vi "Mode 1 - GUI.vi"() -> ()   [LabVIEW 2020]
uses:
  <vilib>/Platform/TimedLoop/XDataNode/timing_clust.ctl
  <vilib>/Platform/TimedLoop/XDataNode/nitl_modes.ctl
  <vilib>/Platform/TimedLoop/XDataNode/wakeup.ctl
  <vilib>/Instr/_visa.llb/VISA Configure Serial Port (Instr).vi
  <vilib>/platform/TimedLoop/XDataNode/XDataNode.xnode
  <vilib>/Platform/TimedLoop/XDataNode/XDNodeRunTimeDep.lvlib
panel:
  in  "byte count":u32=31
  out "Counter Up ?":bool
  in  "Slider 2 Counter":i32
  in  "Slider 1 Counter":i32
  out "Black Workpiece":bool
  out "White Workpiece":bool
  in  "STOP":bool
  in  "VISA resource name":refnum<visa-resource-name>
  out "Report Data":string
  # "TRAINER ARDUINO\nMPS SORTING STATION"
  # "Mechatronics Engineering 2nd Generation\n  Vocational High School 2 Bojonegoro\n2021"
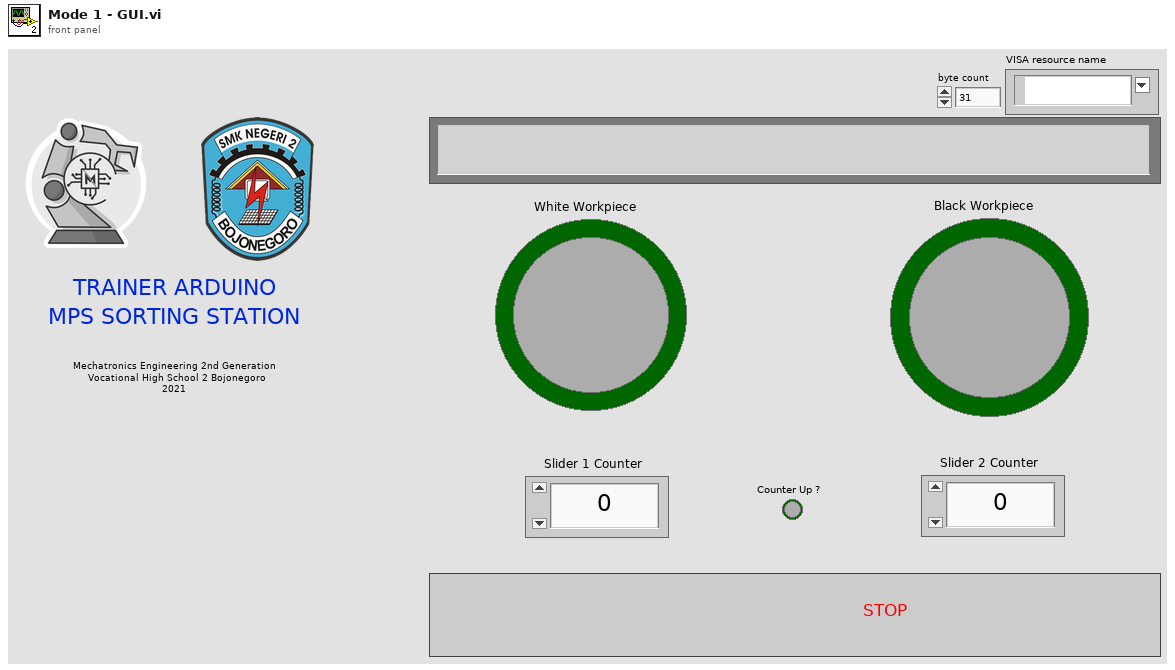
[diagram p1: front panel]
types:
  T1 = typedef "XDNodeRunTimeDep.lvlib/timing_clust.ctl" = cluster{"Expected End [f-1]":u64, "Actual End [f-1]":u64, "Finished Late? [f-1]":bool, "Expected End [i-1]":u64, "Actual End [i-1]":u64, "Finished Late? [i-1]":bool, "Expected Start [i]":u64, "Actual Start [i]":u64, "Expected Start [f]":u64, "Actual Start [f]":u64, "Source Name":string, "Structure Name":string, "Period":i64, "Deadline":i64, "Offset":i64, "Start":i64, "Priority":i32, "Timeout":i32, "Mode":T2, "Wakeup Reason":T3, "Error":errorcluster, "Source Type":string, "Secondary Source Type":string, "Global End Time":u64, "Global Start Time":u64, "Frame Duration":u64, "Iteration Duration":u64, "Assigned CPU":i32, "I/O Scan Engine Mode":u32}
  T2 = typedef "XDNodeRunTimeDep.lvlib/nitl_modes.ctl" = enum32{"No Change", "Process missed periods, maintain original phase", "Discard missed periods, maintain original phase", "Process missed periods, ignore original phase", "Discard missed periods, ignore original phase"}
  T3 = typedef "XDNodeRunTimeDep.lvlib/wakeup.ctl" = enum32{"Normal", "Aborted", "Asynchronous wakeup", "Timing source error", "Timed loop error", "Timeout"}
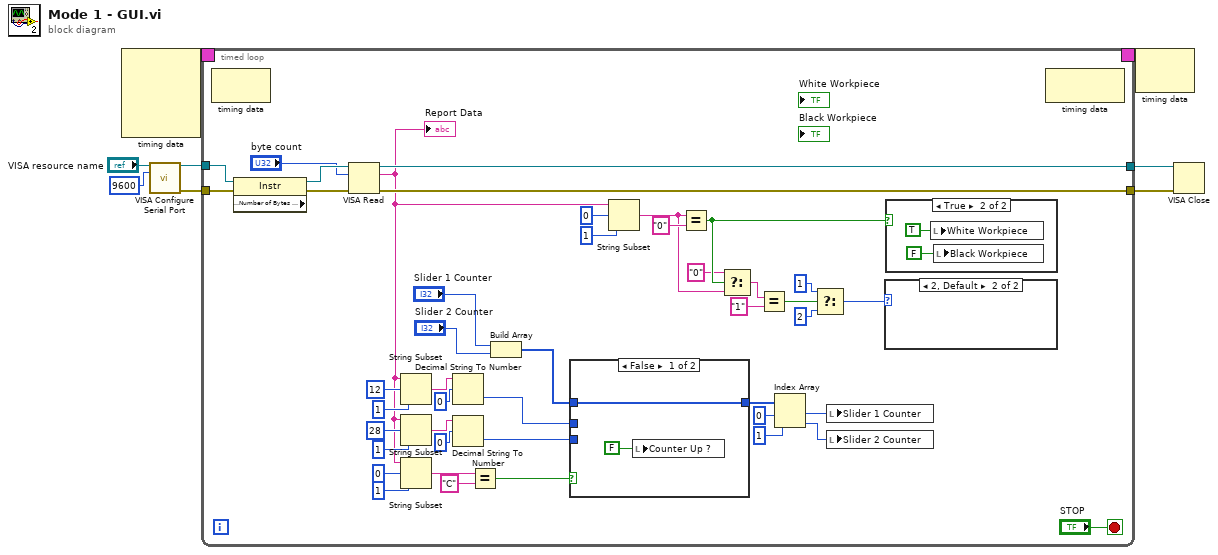
[diagram p0: block diagram]
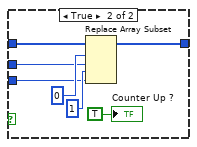
[diagram p2: hidden frame]
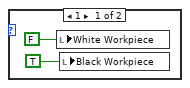
[diagram p3: hidden frame]
diagram:
  n1 = node-c288() -> (w8:T1)  [unwired: 4 in]
  n2 = call-poly "VISA Configure Serial Port"("VISA resource name"="VISA resource name", "baud rate (9600)"=u32 9600) -> ("VISA resource name out"=w6:refnum<visa-resource-name>, "error out"=w5:errorcluster)  [unwired: 12 in]
  n3 = timed-loop {
    timing: w8 -> [_]
    timing-out: [_] -> w7
    tunnel: w6 -> [w52]
    tunnel: w5 -> [w51]
    tunnel: [w48] -> w4
    tunnel: [w47] -> w3
    stop <- "STOP" stop-if-true
    n4 = node-c288() -> ()  [unwired: 1 in, 1 out]
    n5 = property class="Instr" props=["Serial Settings:Number of Bytes at Serial Port"](reference=w52, error in=w51) -> (reference out=w50:refnum<visa-resource-name>, error out=w49:errorcluster)  [unwired: 1 out]
    n6 = VISA Read(VISA resource name=w50, byte count="byte count", error in (no error)=w49) -> (VISA resource name out=w48:refnum<visa-resource-name>, read buffer=w9:string, error out=w47:errorcluster)  [unwired: 1 out]
    "Report Data" <- w9
    n7 = String Subset(string=w9, offset (0)=12, length (rest)=1 ("length (rest)")) -> (substring=w25:string)
    n8 = String Subset(string=w9, offset (0)=28, length (rest)=1 ("length (rest)")) -> (substring=w26:string)
    n9 = String Subset(string=w9, offset (0)=0, length (rest)=1 ("length (rest)")) -> (substring=w29:string)
    n10 = Decimal String To Number(string=w25, offset=0) -> (number=w22:i32)  [unwired: 1 in, 1 out]
    n11 = Decimal String To Number(string=w26, offset=0) -> (number=w21:i32)  [unwired: 1 in, 1 out]
    n12 = Equal?(x=w29, y="C") -> (x = y?=w27:bool)
    n13 = Build Array("Slider 1 Counter", "Slider 2 Counter") -> (w20:i32[])
    n14 = case shown="False" w27 {
      tunnel: w22 -> [_ w59]
      tunnel: w21 -> [_ w58]
      tunnel: w20 -> [w54 w57]
      tunnel: [w54 w56] -> w19
      frame False {
        n15 = local write "Counter Up ?"(FALSE ("Boolean")) -> ()
      }
      frame True {
        n16 = Replace Array Subset(array=w57, new element #1=w59, index #1=0 ("index"), new element #2=w58, index #2=1 ("index")) -> (w56:i32[])
        "Counter Up ?" <- TRUE ("Boolean")
      }
    }
    n17 = String Subset(string=w9, offset (0)=0, length (rest)=1 ("length (rest)")) -> (substring=w10:string)
    n18 = Equal?(x=w10, y="0") -> (x = y?=w43:bool)
    n19 = Select(t="0" ("y"), s=w43, f=w10) -> (s? t:f=w41:string)
    n20 = Equal?(x=w41, y="1") -> (x = y?=w39:bool)
    n21 = Index Array(array=w19, index #1=0 ("index"), index #2=1 ("index")) -> (element #1=w15:i32, element #2=w16:i32)
    n22 = Select(t=1, s=w39, f=2) -> (s? t:f=w38:i32)
    n23 = local write "Slider 1 Counter"(w15) -> ()
    n24 = local write "Slider 2 Counter"(w16) -> ()
    n25 = case shown="2, Default" w38 {
      frame 1 {
        n26 = local write "White Workpiece"(FALSE ("Boolean")) -> ()
        n27 = local write "Black Workpiece"(TRUE ("Boolean")) -> ()
      }
      frame 2, Default {
      }
    }
    n28 = case shown="True" w43 {
      frame False {
      }
      frame True {
        n29 = local write "White Workpiece"(TRUE ("Boolean")) -> ()
        n30 = local write "Black Workpiece"(FALSE ("Boolean")) -> ()
      }
    }
    n31 = node-c288() -> ()  [unwired: 1 in, 1 out]
  }
  n32 = node-c288(w7) -> ()  [unwired: 1 out]
  n33 = VISA Close(VISA resource name=w4, error in (no error)=w3) -> ()  [unwired: 1 out]
